vi "Holoens_GaitDisplay_Simple.vi"() -> ()   [LabVIEW 2016]
uses:
  <vilib>/Utility/miscctls.llb/LV3DPointTypeDef.ctl
  <vilib>/HaroTek/Haro3D/Utilities/3D objects/3D_Quad_class/Panel.lvclass
  C:/Program Files (x86)/National Instruments/LabVIEW 2016/vi.lib/HaroTek/Haro3D/Utilities/3D objects/3D_Shape_class/3D_Shape.lvclass
  <vilib>/picture/3D Picture Control/Object/Add Object (no reference).vi
  <vilib>/HaroTek/Haro3D/Hololens/Hololens_class/Hololens.lvclass
  <vilib>/picture/3D Picture Control/NI_3D Picture Control.lvlib
panel:
  out "3D Picture":refnum<vi>(3d-picture)
  in  "stop":bool
  out "Hololens":bool
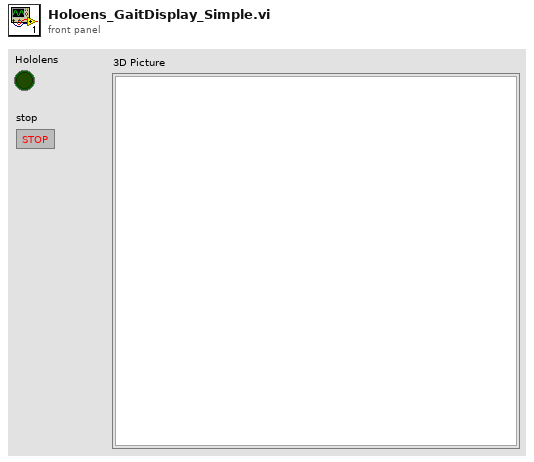
[diagram p1: front panel]
types:
  T1 = typedef "Haro3D.lvlib/Hololens.lvclass/Hololens_event.ctl" = cluster{"Connection":refnum<user-event>, "Data":refnum<user-event>}
  T2 = typedef "LV3DPointTypeDef.ctl" = cluster{"X":sgl, "Y":sgl, "Z":sgl}
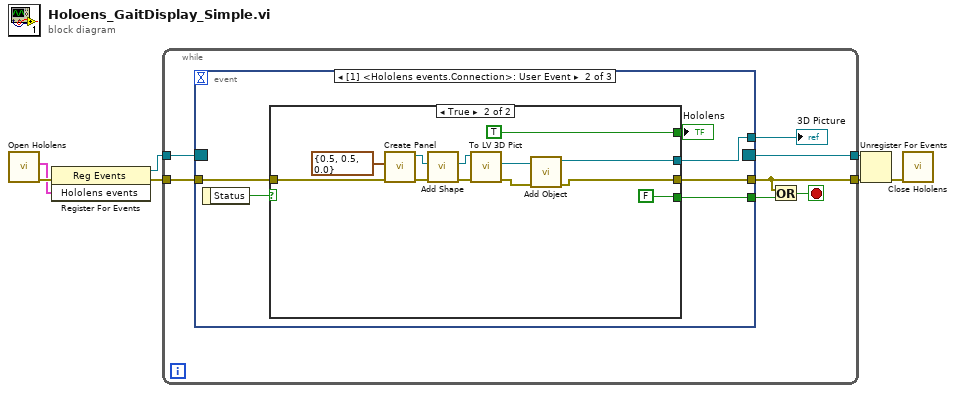
[diagram p0: block diagram]
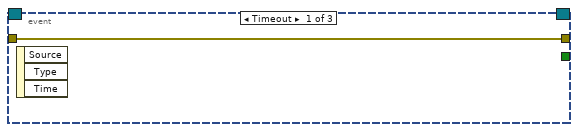
[diagram p2: hidden frame]
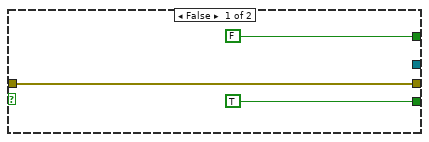
[diagram p3: hidden frame]
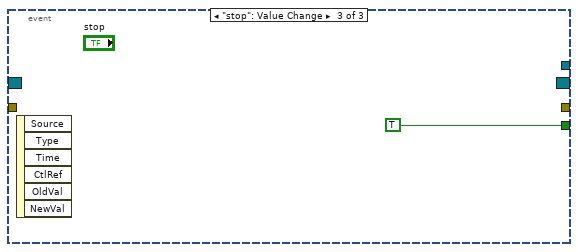
[diagram p4: hidden frame]
diagram:
  n1 = call <vilib>:"Open Hololens.vi"() -> ("error out"=w7:errorcluster, "Hololens events"=w6:T1)  [unwired: 10 in]
  n2 = register-events(error in=w7, w6) -> (reference out=w5:refnum<event-registration>, error out=w2:errorcluster)  [unwired: 1 in]
  n3 = while {
    tunnel: w5 -> [w14]
    tunnel: [w13] -> w3
    tunnel: w2 -> [w12]
    tunnel: [w9] -> w1
    stop <- w10 stop-if-true
    n4 = event shown="[1] <Hololens events.Connection>: User Event" {
      selector: w14 -> [_ _ _]
      dyn-events: [_ _ _] -> w13
      timeout: _ -> [_ _ _]
      tunnel: w12 -> [w15 w20 _]
      tunnel: [w15 w17 _] -> w9
      tunnel: [_ w18 TRUE] -> w11
      tunnel: [_ w16 _] -> w8
      event Timeout {
        n5 = event-data() -> ()  [unwired: 1 in, 3 out]
      }
      event User Event {
        n6 = event-data() -> ("Status"=w21:bool)  [unwired: 1 in]
        n7 = case shown="True" w21 {
          tunnel: w20 -> [w23 w34]
          tunnel: [FALSE TRUE] -> w19
          tunnel: [w23 w27] -> w17
          tunnel: [TRUE FALSE] -> w18
          tunnel: [_ w25] -> w16
          frame False {
          }
          frame True {
            n8 = call <vilib>:"Create Panel.vi"("error in (no error)"=w34, "Dimensions"=T2 {"X"=0.5, "Y"=0.5, "Z"=0.0}) -> ("error out"=w31:errorcluster, "Panel object"=w33:refnum<class "Panel.lvclass">)  [unwired: 8 in]
            n9 = call <vilib>:"Add Shape.vi"("error in (no error)"=w31, "Shape in"=w33) -> ("error out"=w30:errorcluster, "Shape out"=w32:refnum<class "Panel.lvclass">)  [unwired: 7 in, 1 out]
            n10 = call-dynamic "To LV 3D Pict.vi"("error in (no error)"=w30, "reference in"=w32) -> ("error out"=w28:errorcluster, "3D object ref"=w29:refnum<vi>)  [unwired: 7 in, 1 out]
            n11 = call-poly <vilib>:"Add Object.vi"("error in (no error)"=w28, "Scene Object In"=w29) -> ("error out"=w27:errorcluster, "Scene Object Out"=w25:refnum<vi>)  [unwired: 8 in]
          }
        }
        "Hololens" <- w19
      }
      event "stop": Value Change {
        n12 = event-data() -> ()  [unwired: 1 in, 6 out]
      }
    }
    "3D Picture" <- w8
    n13 = Or(x=w9, y=w11) -> (x .or. y?=w10:bool)
  }
  n14 = Unregister For Events(event registration refnum=w3, error in=w1) -> (error out=w4:errorcluster)
  n15 = call <vilib>:"Close Hololens.vi"("error in (no error)"=w4) -> ()  [unwired: 10 in, 1 out]
